vi "markTestActiveT.vi"(8 "error in (no error)":errorcluster, 11 "Model in":refnum<class "Model.lvclass">) -> (0 "error out":errorcluster, 3 "Model out":refnum<class "Model.lvclass">)   [LabVIEW 2013, in "Model.lvclass"]
uses:
  Model.lvclass
  Model.lvclass/Model.ctl
  ApplicationElements/TestMonitor/TestMonitor.lvclass/TestMonitor.ctl
  ApplicationElements/TestMonitor/TestMonitor.lvclass
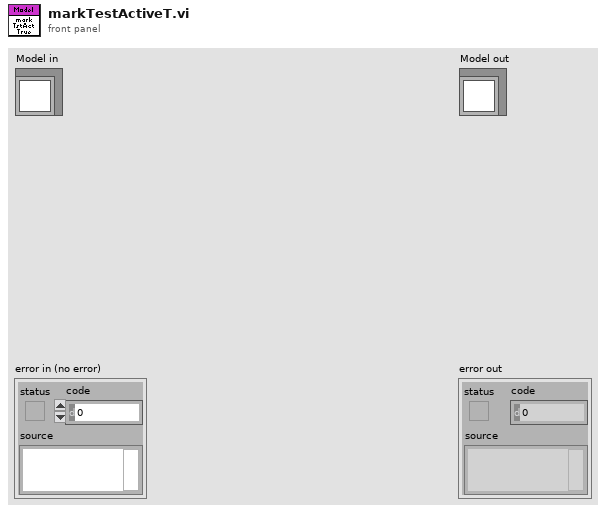
[diagram p1: front panel]
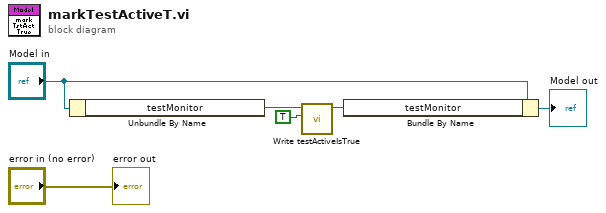
[diagram p0: block diagram]
diagram:
  n1 = Unbundle By Name("Model in") -> ("testMonitor"=w5:refnum<class "TestMonitor.lvclass">)
  n2 = call "Write testActiveIsTrue.vi"("testActiveIsTrue"=TRUE, "TestMonitor in"=w5) -> ("TestMonitor out"=w4:refnum<class "TestMonitor.lvclass">)  [unwired: 9 in]
  n3 = Bundle By Name(cluster="Model in", "testMonitor"=w4) -> (→"Model out":refnum<class "Model.lvclass">)
  "error out" <- "error in (no error)"
